vi "Treat variables only for graph.vi"(7 "Analog values":dbl[](array[numeric]), 11 "error In":errorcluster, 12 "Analog Variable info Settings":T1[](array[typedef]) {"Scaling"."Offset" format="%.5f"; "Scaling"."Gain" format="%.5f"; "Limits and responces"."Limits"."H" format="%.3f"; "Limits and responces"."Limits"."L" format="%.3f"; "Limits and responces"."Limits"."HH" format="%.3f"; "Limits and responces"."Limits"."LL" format="%.3f"}) -> (8 "Analog Values":dbl[](array[numeric]), 15 "error out":errorcluster)   [LabVIEW 2011]
uses:
  User Setting Analog Channel Bg.ctl
  Scaling.ctl
  Alarm Setup Analog.ctl
  Alarm Responce.ctl
  Action List.ctl
  Limits.ctl
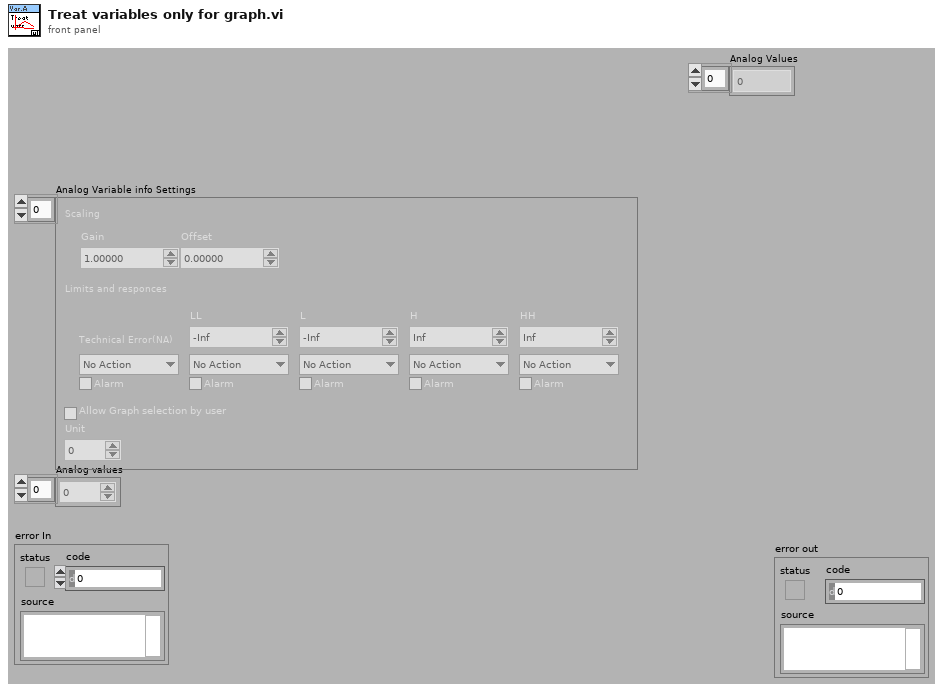
[diagram p1: front panel]
types:
  T1 = typedef "User Setting Analog Channel Bg.ctl" = cluster{"Scaling":T2, "Limits and responces":T3, "Allow Graph selection by user":bool, "Unit":u16}
  T2 = typedef "Scaling.ctl" = cluster{"Gain":dbl, "Offset":dbl}
  T3 = typedef "Alarm Setup Analog.ctl" = cluster{"Technical Error(NA)":T4, "LL":T4, "L":T4, "H":T4, "HH":T4, "Limits":T6}
  T4 = typedef "Alarm Responce.ctl" = cluster{"Action":T5, "Alarm":bool}
  T5 = typedef "Action List.ctl" = enum16{"No Action", "Stop Motor", "Turn Off HV"}
  T6 = typedef "Limits.ctl" = cluster{"LL":dbl, "L":dbl, "H":dbl, "HH":dbl}
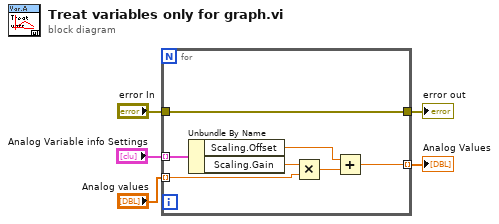
[diagram p0: block diagram]
diagram:
  n1 = for {
    tunnel: "Analog values" -> [w11] mode=indexing
    tunnel: "Analog Variable info Settings" -> [w8] mode=indexing
    tunnel: "error In" -> [w7]
    tunnel: [w7] -> w4
    tunnel: [w6] -> w2 mode=indexing
    n2 = Unbundle By Name(w8) -> ("Scaling.Offset"=w9:dbl, "Scaling.Gain"=w12:dbl)
    n3 = Multiply(x=w12, y=w11) -> (x*y=w10:dbl)
    n4 = Add(x=w9, y=w10) -> (x+y=w6:dbl)
  }
  "Analog Values" <- w2
  "error out" <- w4
